vi "MGCC_MdlMgmt_converttopology.vi"() -> ()   [LabVIEW 2016]
uses:
  Global_MdlMgmt.vi
  <vilib>/imath/engines/lvmath2/RunTimeEngine/IndexRead/NIMS M($,S).vi
  <instcachedir>/0/NIMS M($,S)_3E5749BBB62E49528D4765A77F1F6D98.lvgen/NIMS M($,S)_3E5749BBB62E49528D4765A77F1F6D98_000.vi
  <vilib>/imath/engines/lvmath2/RunTimeEngine/BuiltInFunctions/length/NIMS_length(GV).vi
  <instcachedir>/0/NIMS_length(GV)_08A3D13377FD4E4B96F5795FBF3698FA.lvgen/NIMS_length(GV)_08A3D13377FD4E4B96F5795FBF3698FA_000.vi
  <vilib>/imathl/engines/lvmath/Functions/Error Handling/Create Error.vi
  <vilib>/imath/engines/lvmath2/RunTimeEngine/RangeToken/NIMS_Range_R3 - Integer.vi
  <instcachedir>/0/NIMS_Range_R3 - Integer_A435E2FF893B4C718FD5055FE39FE2F6.lvgen/NIMS_Range_R3 - Integer_A435E2FF893B4C718FD5055FE39FE2F6_000.vi
  <vilib>/imath/engines/lvmath2/RunTimeEngine/CommandStatement/MC_CommandStatement_break.vi
  <vilib>/imath/engines/lvmath2/RunTimeEngine/IndexRead/NIMS M(S,S).vi
  <instcachedir>/0/NIMS M(S,S)_AC51E74150A542F7991B9634C66F3096.lvgen/NIMS M(S,S)_AC51E74150A542F7991B9634C66F3096_000.vi
  <vilib>/imath/engines/lvmath2/RunTimeEngine/IndexRead/NIMS V(S).vi
  <instcachedir>/0/NIMS V(S)_0488751826AF41519A22953C041130DC.lvgen/NIMS V(S)_0488751826AF41519A22953C041130DC_000.vi
  <vilib>/imath/engines/lvmath2/RunTimeEngine/MatrixToken/NIMS_MatrixToken_M_RV.vi
  <instcachedir>/0/NIMS_MatrixToken_M_RV_EE14907D4B194E829889005D2F556E9C.lvgen/NIMS_MatrixToken_M_RV_EE14907D4B194E829889005D2F556E9C_001.vi
  <vilib>/imath/engines/lvmath2/RunTimeEngine/IndexReplace/NIMS M(S,S)=S.vi
  <instcachedir>/0/NIMS M(S,S)=S_98E40400474E4398B113AE20298B4F82.lvgen/NIMS M(S,S)=S_98E40400474E4398B113AE20298B4F82_000.vi
  <vilib>/imath/engines/lvmath2/RunTimeEngine/IndexRead/NIMS M(S,$).vi
  <instcachedir>/0/NIMS M(S,$)_F24F360562DE41D8BE234322A2E15C65.lvgen/NIMS M(S,$)_F24F360562DE41D8BE234322A2E15C65_000.vi
  <vilib>/imath/engines/lvmath2/RunTimeEngine/IndexReplace/NIMS M(S,$)=V.vi
  <instcachedir>/0/NIMS M(S,$)=V_BCCFA522A894489B8FA760383D74A164.lvgen/NIMS M(S,$)=V_BCCFA522A894489B8FA760383D74A164_000.vi
  <vilib>/imath/engines/lvmath2/RunTimeEngine/ErrorHandling/NIMS_Create Error From Enums.vi
  <vilib>/imath/engines/lvmath2/RunTimeEngine/BuiltInFunctions/sortrows/NIMS_sortrows(RM).vi
  <instcachedir>/0/NIMS_sortrows(RM)_A769EDA09CF446F0A0B095F8268DBBEB.lvgen/NIMS_sortrows(RM)_A769EDA09CF446F0A0B095F8268DBBEB_001.vi
  <vilib>/imath/engines/lvmath2/RunTimeEngine/NodeEndStatement/NIMS_NodeEndStatement_Output.vi
  <instcachedir>/0/NIMS_NodeEndStatement_Output_53EC0D466D134D7ABD903AC30B43404B.lvgen/NIMS_NodeEndStatement_Output_53EC0D466D134D7ABD903AC30B43404B_002.vi
  <vilib>/imath/engines/lvmath2/RunTimeEngine/ErrorHandling/NIMS_Finalize Error.vi
  Communication/Global communication output.vi
  <vilib>/imath/engines/lvmath2/RunTimeEngine/BuiltInFunctions/size/NIMS_I32=size(GM,I32).vi
  <instcachedir>/0/NIMS_I32=size(GM,I32)_122058B1B3294FAEA5DC209B92B394E4.lvgen/NIMS_I32=size(GM,I32)_122058B1B3294FAEA5DC209B92B394E4_004.vi
  <vilib>/imath/engines/lvmath2/RunTimeEngine/RangeToken/NIMS_Range_R2 - Integer.vi
  <instcachedir>/0/NIMS_Range_R2 - Integer_89B873E74E6E489885E44F751DD9C6BF.lvgen/NIMS_Range_R2 - Integer_89B873E74E6E489885E44F751DD9C6BF_000.vi
  <instcachedir>/0/NIMS M(S,S)=S_98E40400474E4398B113AE20298B4F82.lvgen/NIMS M(S,S)=S_98E40400474E4398B113AE20298B4F82_002.vi
  <instcachedir>/0/NIMS_NodeEndStatement_Output_53EC0D466D134D7ABD903AC30B43404B.lvgen/NIMS_NodeEndStatement_Output_53EC0D466D134D7ABD903AC30B43404B_005.vi
  <instcachedir>/0/NIMS_NodeEndStatement_Output_53EC0D466D134D7ABD903AC30B43404B.lvgen/NIMS_NodeEndStatement_Output_53EC0D466D134D7ABD903AC30B43404B_010.vi
panel:
  out "BESS":dbl[](array[numeric])
  out "comm_matrix":dbl[][](array[numeric])
  out "Genloc":i32[][](array[numeric])
  out "PVloc":i32[][](array[numeric])
  out "BESSloc":i32[][](array[numeric])
  out "error out 2":errorcluster
  out "PQ BESS location":dbl[](array[numeric])
  out "error out":errorcluster
  in  "Topology":dbl[][](array[numeric])=[[2.0, 1.0, 3.0, 0.0, 100.0, 0.0, 0.0, 0.0, 0.0, 0.0, 0.0, 0.0, 0.0, 0.0, 0.0, 0.0], [3.0, 2.0, 1.0, 0.0, 1.0, 0.0, 0.0, 0.0, 0.0, 0.0, 0.0, 0.0, 0.0, 0.0, 0.0, 0.0], [3.0, 4.0, 1.0, 0.0, 2.0, 0.0, 0.0, 0.0, 0.0, 0.0, 0.0, 0.0, 0.0, 0.0, 0.0, 0.0], [4.0, 5.0, 1.0, 0.0, 4.0, 0.0, 0.0, 0.0, 0.0, 0.0, 0.0, 0.0, 0.0, 0.0, 0.0, 0.0], [4.0, 6.0, 3.0, 0.0, 100.0, 0.0, 0.0, 0.0, 0.0, 0.0, 0.0, 2.0, 1.0, 3.0, 0.0, 100.0], [7.0, 3.0, 1.0, 0.0, 3.0, 0.0, 0.0, 0.0, 0.0, 0.0, 0.0, 3.0, 2.0, 1.0, 0.0, 1.0], [7.0, 8.0, 1.0, 0.0, 5.0, 0.0, 0.0, 0.0, 0.0, 0.0, 0.0, 3.0, 4.0, 1.0, 0.0, 2.0], [9.0, 7.0, 1.0, 0.0, 6.0, 0.0, 0.0, 0.0, 0.0, 0.0, 0.0, 4.0, 5.0, 1.0, 0.0, 4.0], [10.0, 9.0, 1.0, 0.0, 7.0, 0.0, 0.0, 0.0, 0.0, 0.0, 0.0, 4.0, 6.0, 3.0, 0.0, 100.0], [10.0, 13.0, 3.0, 0.0, 100.0, 0.0, 0.0, 0.0, 0.0, 0.0, 0.0, 7.0, 3.0, 1.0, 0.0, 3.0], [10.0, 12.0, 3.0, 0.0, 100.0, 0.0, 0.0, 0.0, 0.0, 0.0, 0.0, 8.0, 7.0, 1.0, 0.0, 5.0], [10.0, 11.0, 1.0, 0.0, 8.0, 0.0, 0.0, 0.0, 0.0, 0.0, 0.0, 9.0, 7.0, 1.0, 0.0, 6.0], [11.0, 14.0, 3.0, 0.0, 100.0, 0.0, 0.0, 0.0, 0.0, 0.0, 0.0, 10.0, 9.0, 1.0, 0.0, 7.0], [0.0, 0.0, 0.0, 0.0, 0.0, 0.0, 0.0, 0.0, 0.0, 0.0, 0.0, 10.0, 13.0, 2.0, 0.0, 100.0], [0.0, 0.0, 0.0, 0.0, 0.0, 0.0, 0.0, 0.0, 0.0, 0.0, 0.0, 10.0, 12.0, 2.0, 0.0, 100.0], [0.0, 0.0, 0.0, 0.0, 0.0, 0.0, 0.0, 0.0, 0.0, 0.0, 0.0, 10.0, 11.0, 1.0, 0.0, 8.0], [0.0, 0.0, 0.0, 0.0, 0.0, 0.0, 0.0, 0.0, 0.0, 0.0, 0.0, 11.0, 14.0, 3.0, 0.0, 100.0]]
  out "Equal_M":dbl[][](array[numeric])
  out "Microgrid Topology Overall":dbl[][](array[numeric])
  out "array w/ subset deleted":dbl[][](array[numeric])
  out "Topology_identification":dbl[][](array[numeric])
  out "Topology_overall":dbl[][](array[numeric])
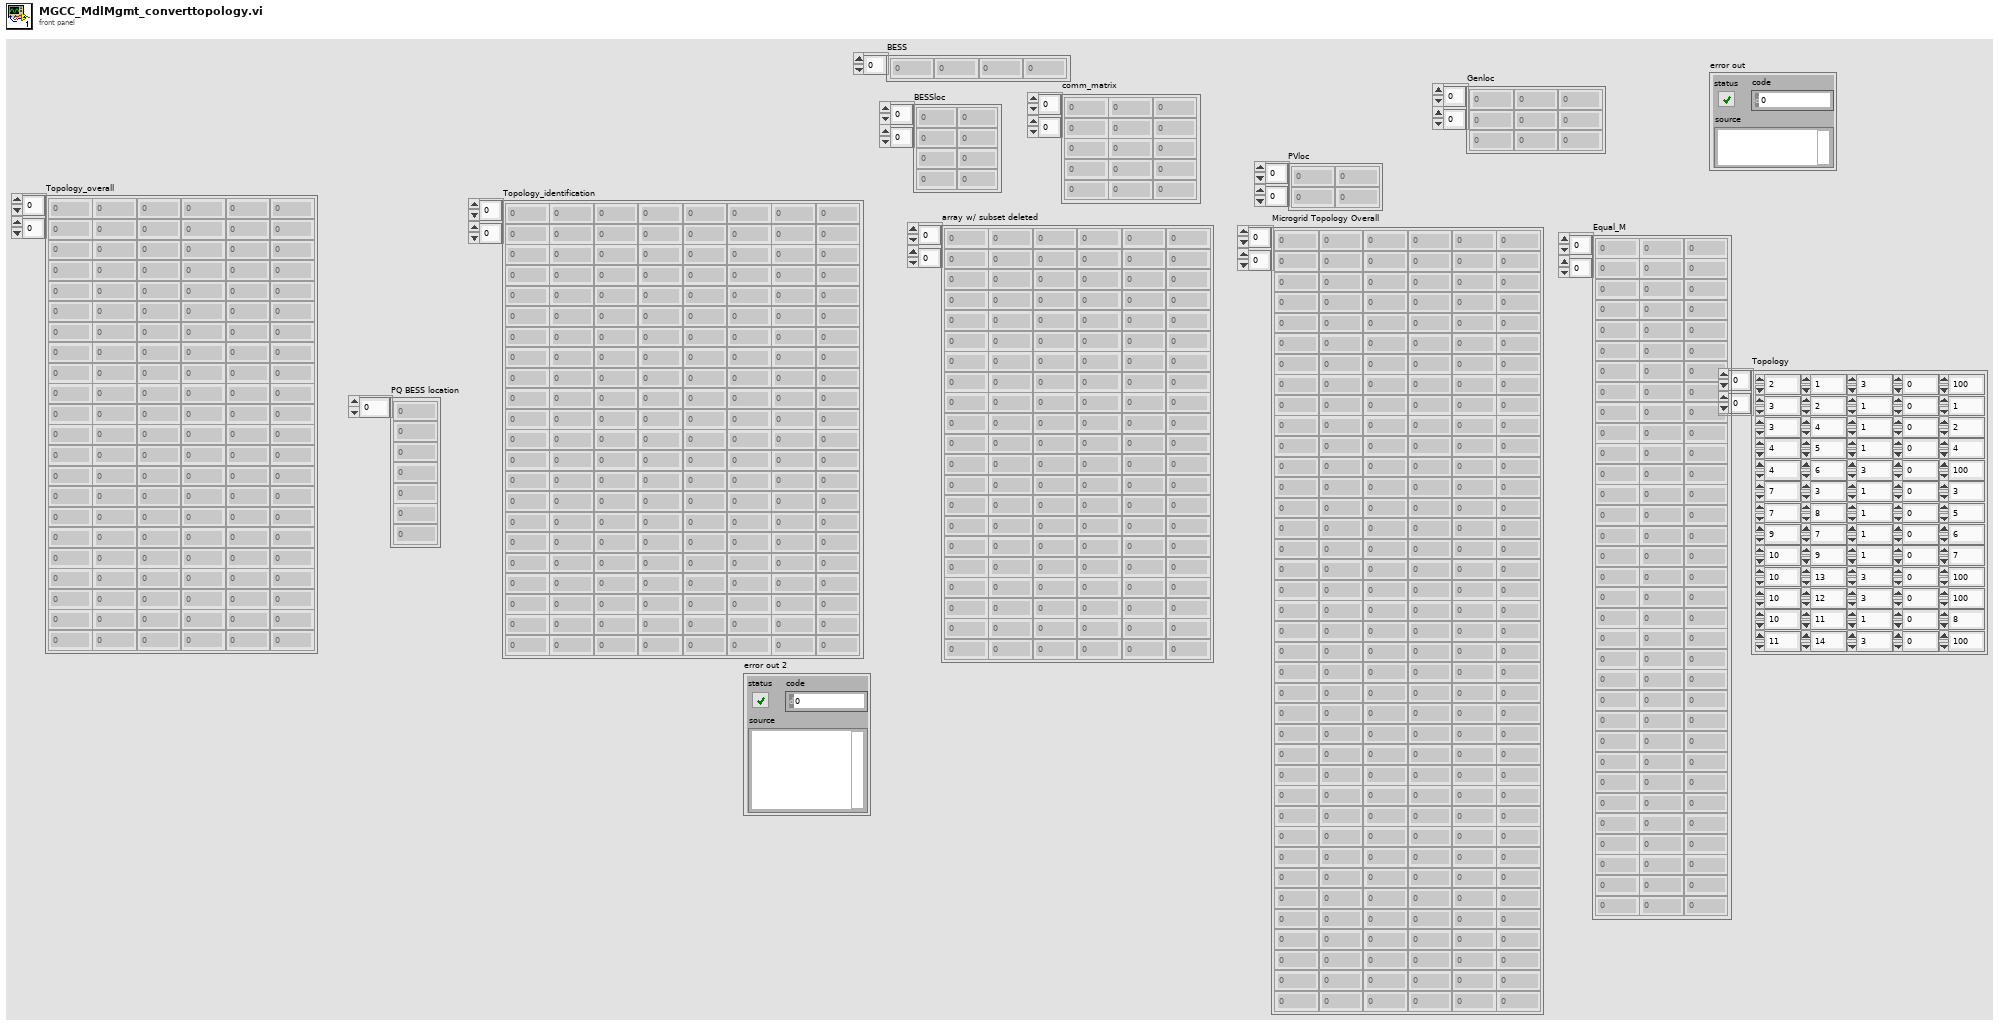
[diagram p1: front panel]
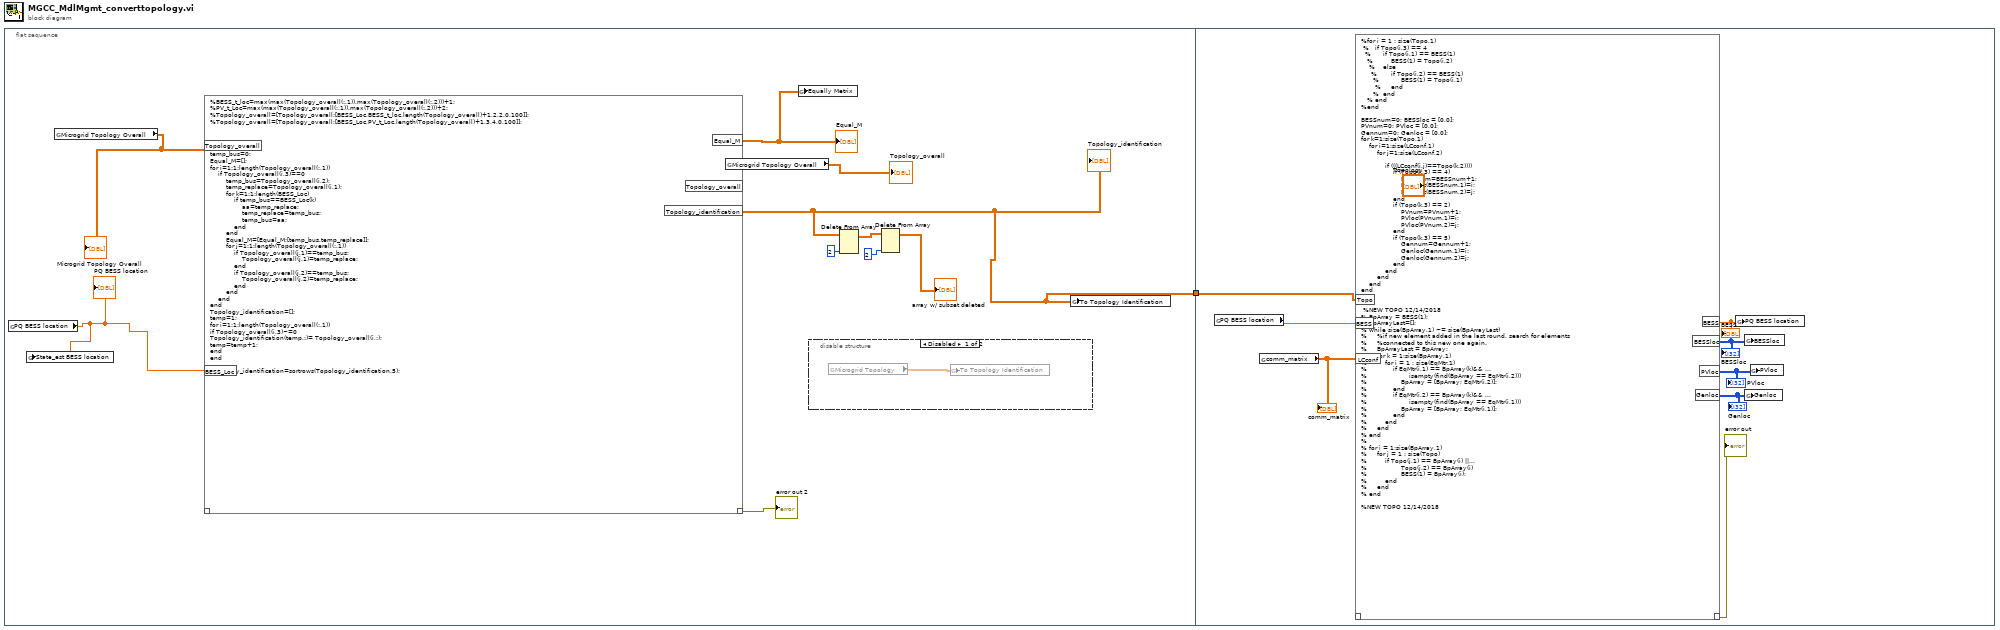
[diagram p0: block diagram]
diagram:
  n1 = flat-sequence {
    tunnel: [w2] -> w1
    tunnel: w1 -> [w678]
    frame #0 {
      n2 = global read "Global_MdlMgmt.vi" "PQ BESS location"() -> (w3:dbl[])
      "PQ BESS location" <- w3
      n3 = global write "Global_MdlMgmt.vi" "State_est BESS location"(w3) -> ()
      n4 = global read "Global_MdlMgmt.vi" "Microgrid Topology Overall"() -> (w11:dbl[][])
      "Microgrid Topology Overall" <- w11
      n5 = mathscript code="%BESS_t_loc=max(max(Topology_overall(:,1)),max(Topology_overall(:,2)))+1;\n%PV_t_Loc=max(max(Topology_overall(:,1)),max(Topology_overall(:,2)))+2;\n%Topology_overall=[Topology_overall;[BESS_Loc,BESS_t_loc,length(Topology_overall)+1,2,2,0,100]];\n%Topology_overall=[Topology_overall;[BESS_Loc,PV_t_Loc,length(Topology_overall)+1,3,4,0,100]];\n\n\n\n\ntemp_bus=0;\nEqual_M=[];\nfor i=1:1:length(Topology_overall(:,1))\n    if Topology_overall(i,3)==0\n        temp_bus=Topology_overall(i,2);\n        temp_replace=Topology_overall(i,1);\n        for k=1:1:length(BESS_Loc)\n            if temp_bus==BESS_Loc(k)\n                aa=temp_replace;\n                temp_replace=temp_bus;\n                temp_bus=aa;\n            end\n        end\n        Equal_M=[Equal_M;[temp_bus,temp_replace]];\n        for j=1:1:length(Topology_overall(:,1))\n            if Topology_overall(j,1)==temp_bus;\n                Topology_overall(j,1)=temp_replace;\n            end\n            if Topology_overall(j,2)==temp_bus;\n                Topology_overall(j,2)=temp_replace;\n            end\n        end\n    end\nend\nTopology_identification=[];\ntemp=1;\nfor i=1:1:length(Topology_overall(:,1))\nif Topology_overall(i,3)~=0\nTopology_identification(temp,:)= Topology_overall(i,:);\ntemp=temp+1;\nend\nend\n\nTopology_identification=sortrows(Topology_identification,5);"("Topology_overall"=w11, "BESS_Loc"=w3) -> ("??"=→"error out 2":errorcluster, "Topology_identification"=w2:dbl[][], "Equal_M"=w7:dbl[][])  [unwired: 1 in, 1 out]
      "Topology_identification" <- w2
      "Equal_M" <- w7
      n6 = global read "Global_MdlMgmt.vi" "Microgrid Topology Overall"() -> (→"Topology_overall":dbl[][])
      n7 = global write "Global_MdlMgmt.vi" "Equally Metrix"(w7) -> ()
      n8 = disable-structure shown="Disabled" {
        frame Disabled {
          n9 = global read "Global_MdlMgmt.vi" "Microgrid Topology"() -> (w12:dbl[][])
          n10 = global write "Global_MdlMgmt.vi" "To Topology Identification"(w12) -> ()
        }
        frame Enabled {
        }
      }
      n11 = Delete From Array(array=w2, index (col)=2 ("disabled index (col)")) -> (array with subset deleted=w9:dbl[][])  [unwired: 2 in, 1 out]
      n12 = Delete From Array(array=w9, index (col)=2 ("disabled index (col)")) -> (array with subset deleted=→"array w/ subset deleted":dbl[][])  [unwired: 2 in, 1 out]
      n13 = global write "Global_MdlMgmt.vi" "To Topology Identification"(w2) -> ()
    }
    frame #1 {
      n14 = global read "Global_MdlMgmt.vi" "PQ BESS location"() -> (w681:dbl[])
      n15 = global read "Global communication output.vi" "comm_matrix"() -> (w677:dbl[][])
      "comm_matrix" <- w677
      n16 = mathscript code="%for i = 1 : size(Topo,1)\n %   if Topo(i,3) == 4\n  %      if Topo(i,1) == BESS(1)\n   %         BESS(1) = Topo(i,2)\n    %    else\n     %       if Topo(i,2) == BESS(1)\n      %           BESS(1) = Topo(i,1)\n       %     end\n      %  end        \n   % end\n%end\n\nBESSnum=0; BESSloc = [0,0];\nPVnum=0; PVloc = [0,0];\nGennum=0; Genloc = [0,0];\nfor k=1:size(Topo,1)\n    for i=1:size(LCconf,1)\n        for j=1:size(LCconf,2)\n\n            if (((LCconf(i,j)==Topo(k,2))))\n                if (Topo(k,3) == 4)\n                    BESSnum=BESSnum+1;\n                    BESSloc(BESSnum,1)=i;\n                    BESSloc(BESSnum,2)=j;\n                end\n                if (Topo(k,3) == 2)\n                    PVnum=PVnum+1;\n                    PVloc(PVnum,1)=i;\n                    PVloc(PVnum,2)=j;\n                end\n                if (Topo(k,3) == 5)\n                    Gennum=Gennum+1;\n                    Genloc(Gennum,1)=i;\n                    Genloc(Gennum,2)=j;\n                end\n            end\n        end\n    end\nend\n\n\n %NEW TOPO 12/14/2018\n% BpArray = BESS(1);\n% BpArrayLast=[];\n% while size(BpArray,1) ~= size(BpArrayLast)\n%     %if new element added in the last round, search for elements\n%     %connected to this new one again.\n%     BpArrayLast = BpArray;\n%     for k = 1:size(BpArray,1)\n%         for i = 1 : size(EqMtr,1)\n%             if EqMtr(i,1) == BpArray(k)&& ...\n%                     isempty(find(BpArray == EqMtr(i,2)))\n%                 BpArray = [BpArray; EqMtr(i,2)];\n%             end\n%             if EqMtr(i,2) == BpArray(k)&& ...\n%                     isempty(find(BpArray == EqMtr(i,1)))\n%                 BpArray = [BpArray; EqMtr(i,1)];\n%             end\n%         end\n%     end\n% end\n% \n% for i = 1:size(BpArray,1)\n%     for j = 1 : size(Topo)\n%         if Topo(j,1) == BpArray(i) ||...\n%                 Topo(j,2) == BpArray(i)\n%                 BESS(1) = BpArray(i);\n%         end\n%     end\n% end\n\n%NEW TOPO 12/14/2018"("Topo"=w678, "BESS"=w681, "LCconf"=w677) -> ("??"=→"error out":errorcluster, "BESS"=w679:dbl[], "BESSloc"=w676:i32[][], "PVloc"=w675:i32[][], "Genloc"=w674:i32[][])  [unwired: 1 in]
      "BESSloc" <- w676
      "PVloc" <- w675
      "Genloc" <- w674
      "BESS" <- w679
      n17 = global write "Global_MdlMgmt.vi" "PQ BESS location"(w679) -> ()
      n18 = global write "Global_MdlMgmt.vi" "BESSloc"(w676) -> ()
      n19 = global write "Global_MdlMgmt.vi" "Genloc"(w674) -> ()
      n20 = global write "Global_MdlMgmt.vi" "PVloc"(w675) -> ()
    }
  }
